vi "DevSP.vi"(7 "LabVIEW Web Service Request":refnum<class "Web Request.lvclass">, 10 "SP":dbl, 11 "DevID":string) -> ()   [LabVIEW 2014]
uses:
  <vilib>/wsapi/Web Request.lvclass
  Controller/Messages/Update Device Setpoint MSG/Update Device Setpoint.lvclass
  Controller/Messages/Update Device Setpoint MSG/Update Device Setpoint.lvclass/Update Device Setpoint.ctl
  Controller/Messages/Update Device Setpoint MSG/Write DevID.vi
  Controller/Messages/Update Device Setpoint MSG/Write SP.vi
  Controller/Controller.lvclass
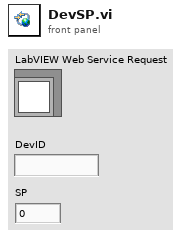
[diagram p1: front panel]
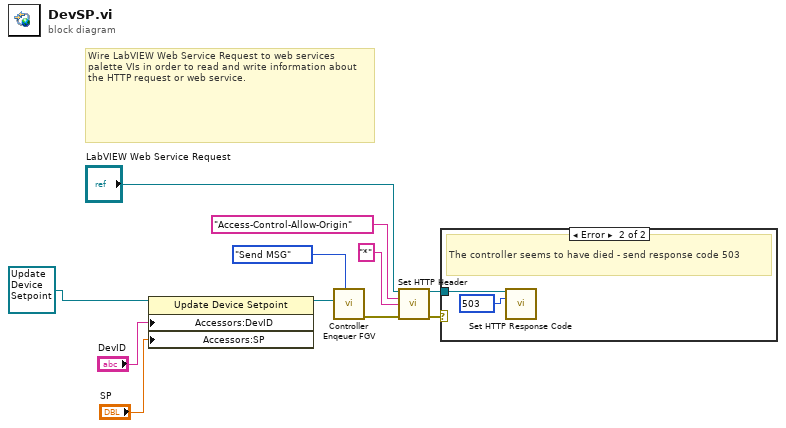
[diagram p0: block diagram]
diagram:
  # "Wire LabVIEW Web Service Request to web services palette VIs in order to read and write information about the HTTP request or web service."
  n1 = property class="Update Device Setpoint"(reference=refnum<class "Update Device Setpoint.lvclass"> refnum ("Controller.lvlib:Update Device Setpoint"), "Accessors:DevID"="DevID", "Accessors:SP"="SP") -> (reference out=w3:refnum<class "Update Device Setpoint.lvclass">)  [unwired: 1 in, 1 out]
  n2 = call "Controller Enqeuer FGV.vi"("State"=enum16{"Store", "Send MSG"}."Send MSG", "MSG"=w3) -> ("error out"=w2:errorcluster)  [unwired: 9 in]
  n3 = call <vilib>:"Set HTTP Header.vi"("LabVIEW Web Service Request"="LabVIEW Web Service Request", "header"="Access-Control-Allow-Origin", "header value"="*", "error in (no error)"=w2) -> ("LabVIEW Web Service Request out"=w8:refnum<class "Web Request.lvclass">, "error out"=w7:errorcluster)  [unwired: 10 in]
  n4 = case shown="Error" w7 {
    tunnel: w8 -> [_ w12]
    frame No Error {
    }
    frame Error {
      w13 = 503 items=["100"=100, "101"=101, "200"=200, "201"=201, "202"=202, "203"=203, "204"=204, "205"=205, "206"=206, "300"=300, "301"=301, "302"=302, "303"=303, "304"=304, "305"=305, "306"=306, "307"=307, "400"=400, "401"=401, "402"=402, "403"=403, "404"=404, "405"=405, "406"=406, "407"=407, "408"=408, "409"=409, "410"=410, "411"=411, "412"=412, "413"=413, "414"=414, "415"=415, "416"=416, "417"=417, "500"=500, "501"=501, "502"=502, "503"=503, "504"=504, "505"=505] ("response code (200)")
      # "The controller seems to have died - send response code 503"
      n5 = call <vilib>:"Set HTTP Response Code.vi"("LabVIEW Web Service Request"=w12, "response code (200)"=w13) -> ()  [unwired: 12 in, 2 out]
    }
  }
